vi "AddDefaultFPModules.vi"(5 "modules":T1[](array[typedef])=[{"Python module"="multiprocessing", "Python module  name"="mp"}, {"Python module"="threading", "Python module  name"=""}, {"Python module"="pyVI.FP.lvFrontPanel", "Python module  name"="lvFP"}, {"Python module"="pyVI.VI.lvDataTypes", "Python module  name"="lvDT"}, {"Python module"="pyVI.VI.lvApplication", "Python module  name"="lvApp"}, {"Python module"="tkinter", "Python module  name"="tk"}, {"Python module"="BlockDiagram", "Python module  name"="BD"}], 6 "error in":errorcluster, 9 "PythonConverter_GUI in":refnum<class "PythonConverter_GUI.lvclass">) -> (0 "error out":errorcluster, 3 "PythonConverter_GUI out":refnum<class "PythonConverter_GUI.lvclass">)   [LabVIEW 2014, in "Raspberry Pi Compatible Compiler for LabVIEW.lvlib" / "PythonConverter_GUI.lvclass"]
uses:
  PythonConverter_GUI.lvclass
  TypeDefs/PythonModuleTD.ctl
  PythonConverter_GUI.lvclass/PythonConverter_GUI.ctl
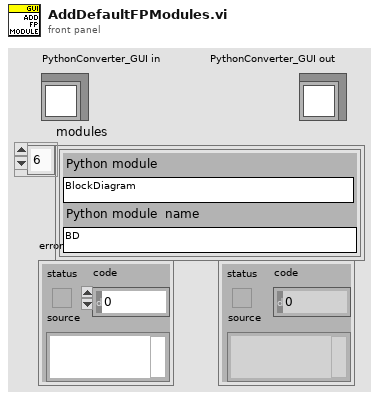
[diagram p1: front panel]
types:
  T1 = typedef "Raspberry Pi Compatible Compiler for LabVIEW.lvlib/PythonConverter_GUI.lvclass/PythonModuleTD.ctl" = cluster{"Python module":string, "Python module  name":string}
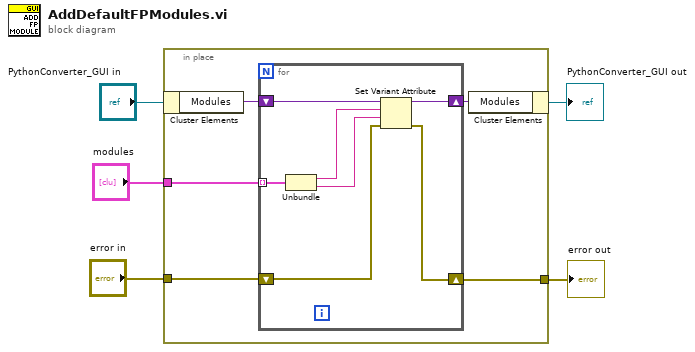
[diagram p0: block diagram]
diagram:
  n1 = in-place {
    in-place-border: "error in" -> [w8]
    in-place-border: [w7] -> w2
    in-place-border: "modules" -> [w6]
    n2 = in-place-cluster #1("PythonConverter_GUI in") -> ("Modules"=w10:variant)
    n3 = for {
      shift-right: [w16] -> w9
      shift-left: w10 -> [w17]
      shift-right: [w14] -> w7
      shift-left: w8 -> [w15]
      tunnel: w6 -> [w13] mode=indexing
      n4 = Unbundle(w13) -> ("Python module"=w12:string, "Python module  name"=w11:string)
      n5 = Set Variant Attribute(Variant=w17, name=w12, value=w11, error in=w15) -> (Variant out=w16:variant, error out=w14:errorcluster)  [unwired: 1 out]
    }
    n6 = in-place-cluster #1("Modules"=w9) -> (→"PythonConverter_GUI out":refnum<class "PythonConverter_GUI.lvclass">)
  }
  "error out" <- w2
